vi "Meas Proc QWTB String to Table Writter.vi"(7 "param table ref":refnum<vi>, 8 "error in":errorcluster, 9 "force data update? (False)":bool, 10 "signaling update? (True)":bool=TRUE, 11 "content csv string":string) -> (0 "error out":errorcluster)   [LabVIEW 2013]
doc: "This VI will take spreadsheet string table and writes it to the referenced table. It sets formats if the table headers to bold."
uses:
  <vilib>/Utility/miscctls.llb/LVRowAndColumnTypeDef.ctl
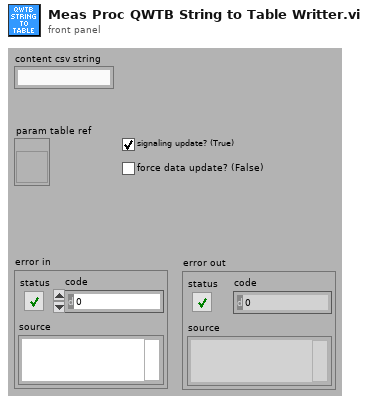
[diagram p1: front panel]
types:
  T1 = typedef "LVRowAndColumnTypeDef.ctl" = cluster{"Row":i32, "Column":i32}
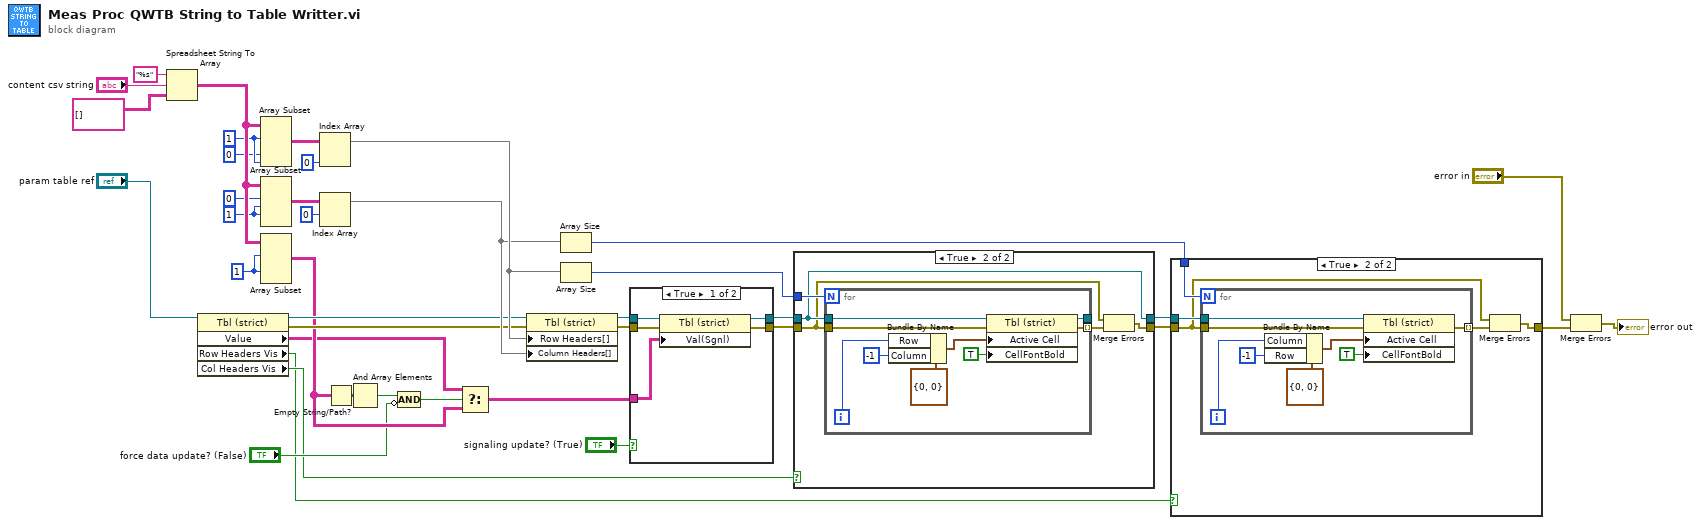
[diagram p0: block diagram]
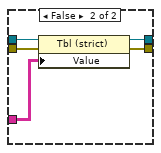
[diagram p4: hidden frame]
diagram:
  w26 = 1 ("index")
  w27 = 1 ("index")
  w21 = 1 ("disabled index (col)")
  n1 = Spreadsheet String To Array(format string="%s", spreadsheet string="content csv string", array type (2D Dbl)=string[][] []) -> (array=w37:string[][])  [unwired: 1 in]
  n2 = property class="Tbl (strict)"(reference="param table ref") -> (reference out=w16:refnum<vi>, error out=w18:errorcluster, "Value"=w13:string[][], "Row Headers Vis"=w1:bool, "Col Headers Vis"=w2:bool)  [unwired: 1 in]
  n3 = Array Subset(array=w37, index (row)=w26, index (col)=0 ("index"), length (col)=w26) -> (w32:string[][])  [unwired: 1 in]
  n4 = Array Subset(array=w37, index (row)=0 ("disabled index (col)"), length (row)=w21, index (col)=w21) -> (w30:string[][])  [unwired: 1 in]
  n5 = Array Subset(array=w37, index (row)=w27, index (col)=w27) -> (w14:string[][])  [unwired: 2 in]
  n6 = Index Array(array=w32, index (col)=0 ("disabled index (col)")) -> (element=w24:string[])  [unwired: 1 in]
  n7 = Index Array(array=w30, index (row)=0) -> (element=w22:string[])  [unwired: 1 in]
  n8 = Empty String/Path?(string/path=w14) -> (empty?=w15:bool[][])
  n9 = And Array Elements(Boolean array=w15) -> (logical AND=w4:bool)
  n10 = Compound Arithmetic op=AND(w4, invert "force data update? (False)") -> (w5:bool)
  n11 = Select(t=w13, s=w5, f=w14) -> (s? t:f=w7:string[][])
  n12 = property class="Tbl (strict)"(reference=w16, error in=w18, "Row Headers[]"=w24, "Column Headers[]"=w22) -> (reference out=w8:refnum<vi>, error out=w11:errorcluster)
  n13 = Array Size(array=w22) -> (size(s)=w29:i32)
  n14 = Array Size(array=w24) -> (size(s)=w31:i32)
  n15 = case shown="True" "signaling update? (True)" {
    tunnel: w11 -> [w44 w49]
    tunnel: [w43 w48] -> w10
    tunnel: [w42 w47] -> w9
    tunnel: w8 -> [w41 w46]
    tunnel: w7 -> [w40 w45]
    frame True {
      n16 = property class="Tbl (strict)"(reference=w41, error in=w44, "Val(Sgnl)"=w40) -> (reference out=w42:refnum<vi>, error out=w43:errorcluster)
    }
    frame False {
      n17 = property class="Tbl (strict)"(reference=w46, error in=w49, "Value"=w45) -> (reference out=w47:refnum<vi>, error out=w48:errorcluster)
    }
  }
  n18 = case shown="True" w2 {
    tunnel: [w51 w55] -> w35
    tunnel: [w50 w53] -> w34
    tunnel: w31 -> [_ w54]
    tunnel: w10 -> [w51 w52]
    tunnel: w9 -> [w50 w53]
    frame False {
    }
    frame True {
      n19 = for {
        N: w54 -> [_]
        tunnel: w52 -> [w65]
        tunnel: [w59] -> w56 mode=indexing
        tunnel: w53 -> [w58]
        tunnel: [w57] -> _
        i -> [w61]
        n20 = Bundle By Name(cluster=T1 {"Row"=0, "Column"=0} ("Active Cell:Active Cell"), "Row"=w61, "Column"=-1) -> (w64:T1)
        n21 = property class="Tbl (strict)"(reference=w58, error in=w65, "Active Cell"=w64, "CellFontBold"=TRUE ("Active Cell:Cell Font:Bold")) -> (reference out=w57:refnum<vi>, error out=w59:errorcluster)
      }
      n22 = Merge Errors(w52, w56) -> (w55:errorcluster)
    }
  }
  n23 = case shown="True" w1 {
    tunnel: [w66 w68] -> w36
    tunnel: w35 -> [w66 w67]
    tunnel: w34 -> [_ w70]
    tunnel: w29 -> [_ w69]
    frame False {
    }
    frame True {
      n24 = for {
        N: w69 -> [_]
        tunnel: w67 -> [w79]
        tunnel: [w73] -> w71 mode=indexing
        tunnel: w70 -> [w72]
        i -> [w75]
        n25 = Bundle By Name(cluster=T1 {"Row"=0, "Column"=0} ("Active Cell:Active Cell"), "Column"=w75, "Row"=-1 ("Column")) -> (w78:T1)
        n26 = property class="Tbl (strict)"(reference=w72, error in=w79, "Active Cell"=w78, "CellFontBold"=TRUE ("Active Cell:Cell Font:Bold")) -> (error out=w73:errorcluster)  [unwired: 1 out]
      }
      n27 = Merge Errors(w67, w71) -> (w68:errorcluster)
    }
  }
  n28 = Merge Errors("error in", w36) -> (→"error out":errorcluster)
